vi "Writer data.vi"(8 "error in":errorcluster caption="错误输入（无错误）", 9 "数据输入":string[](array[string])=["TBOX", "7900020-CC102", "1", "1", "1", "2018/11/14 14:56:51 ", "1", "1", "1"], 11 "Slot":T1) -> (0 "error out":errorcluster caption="错误输出", 2 "Pass?":bool, 3 "添加的数组":string[][](array[string]))   [LabVIEW 2013]
uses:
  SystemCode/SysControl/Slot.ctl
  <vilib>/Utility/NIReport.llb/NI_report.lvclass
  <vilib>/addons/_office/excel.llb/Excel Get Data ([str]).vi
  <vilib>/addons/_office/excel.llb/Excel Easy Table (str).vi
  <vilib>/addons/_office/NI_ReportGenerationToolkit.lvlib
  <vilib>/Utility/NIReport.llb/Excel/NI_Excel.lvclass
panel:
  out "exists?":bool caption="文件或文件夹存在？"
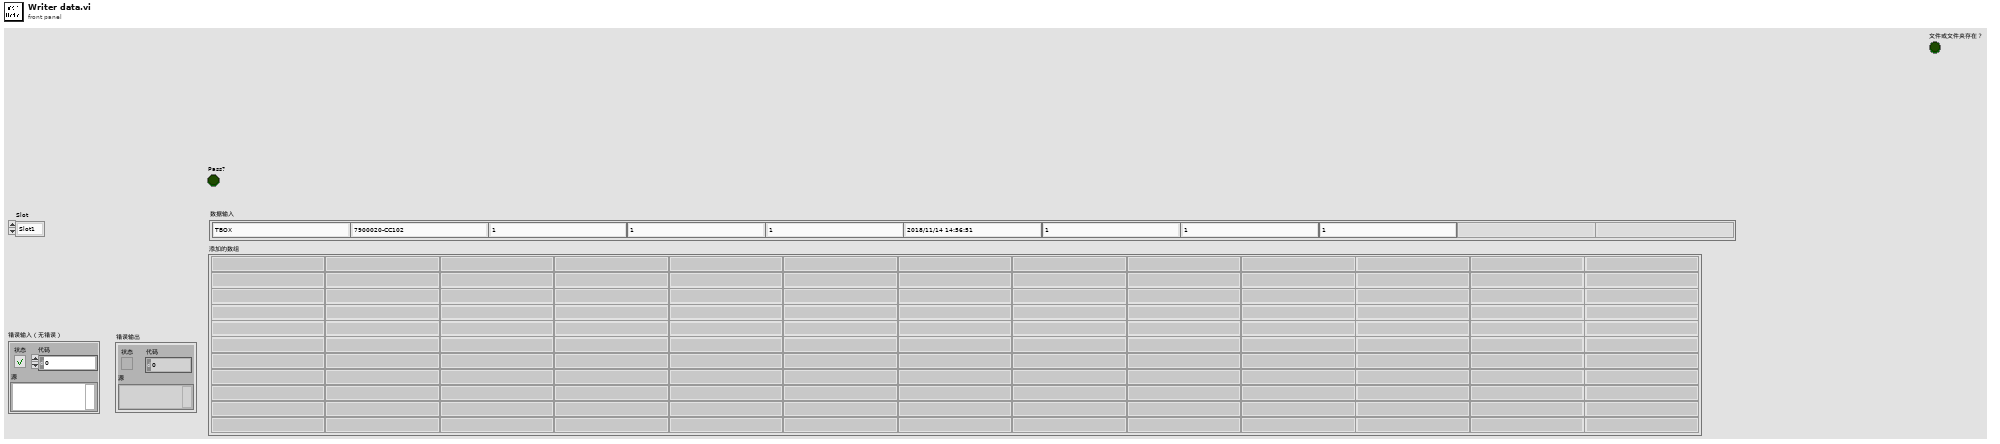
[diagram p1: front panel]
types:
  T1 = typedef "Slot.ctl" = enum16{"Slot1", "Slot2", "Slot3", "Slot4"}
  T2 = enum16{"Standard Report", "HTML", "Word", "Excel"}
  T3 = enum16{"maximized", "minimized", "normal", "no change"}
  T4 = enum32{"invalid app kind", "Development System", "Run Time System", "Student Edition", "Embedded LabVIEW", "Evaluation", "Custom"}
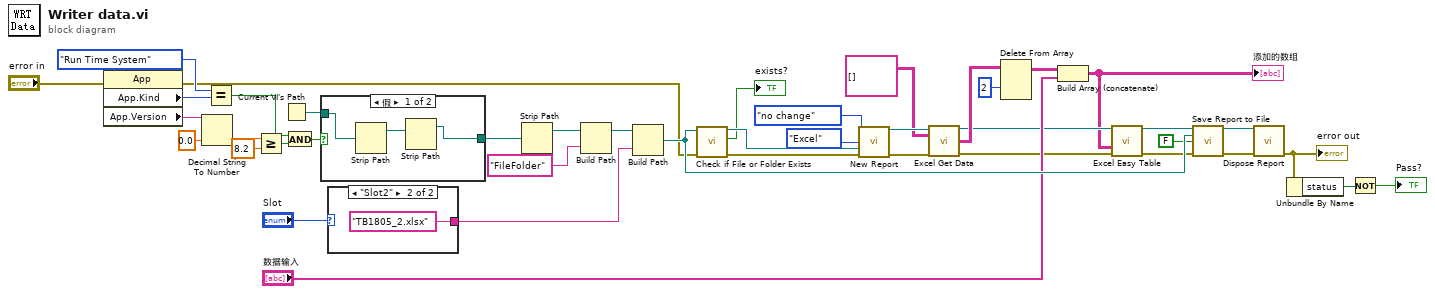
[diagram p0: block diagram]
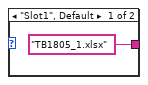
[diagram p2: hidden frame]
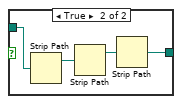
[diagram p3: hidden frame]
diagram:
  n1 = property class="App"(error in="error in") -> (error out=w4:errorcluster, "App.Kind"=w42:T4, "App.Version"=w40:string)  [unwired: 1 in, 1 out]
  n2 = Decimal String To Number(string=w40, default (0L)=0.0 ("数值")) -> (number=w39:dbl)  [unwired: 1 in, 1 out]
  n3 = Equal?(x=T4."Run Time System" ("应用程序:类别"), y=w42) -> (x = y?=w36:bool)
  n4 = Greater Or Equal?(x=w39, y=8.2) -> (x >= y?=w35:bool)
  n5 = Current VI's Path() -> (path=w33:path)
  n6 = And(x=w36, y=w35) -> (x .and. y?=w34:bool)
  n7 = case shown="假" w34 {
    tunnel: w33 -> [w45 w49]
    tunnel: [w43 w46] -> w32
    frame False {
      n8 = Strip Path(path=w45) -> (stripped path=w44:path)  [unwired: 1 out]
      n9 = Strip Path(path=w44) -> (stripped path=w43:path)  [unwired: 1 out]
    }
    frame True {
      n10 = Strip Path(path=w49) -> (stripped path=w48:path)  [unwired: 1 out]
      n11 = Strip Path(path=w48) -> (stripped path=w47:path)  [unwired: 1 out]
      n12 = Strip Path(path=w47) -> (stripped path=w46:path)  [unwired: 1 out]
    }
  }
  n13 = case shown="\"Slot2\"" "Slot" {
    tunnel: ["TB1805_1.xlsx" ("名称或相对路径") "TB1805_2.xlsx" ("名称或相对路径")] -> w8
    frame "Slot1", Default {
    }
    frame "Slot2" {
    }
  }
  n14 = Strip Path(path=w32) -> (stripped path=w31:path)  [unwired: 1 out]
  n15 = Build Path(base path=w31, name or relative path="FileFolder" ("名称或相对路径")) -> (appended path=w6:path)
  n16 = Build Path(base path=w6, name or relative path=w8) -> (appended path=w20:path)
  n17 = call <vilib>:"Check if File or Folder Exists.vi"("error in (no error)"=w4, "path"=w20) -> ("error out"=w27:errorcluster, "file or folder exists?"=→"exists?":bool, "dup path"=w30:path)  [unwired: 7 in]
  n18 = call <vilib>:"New Report.vi"("window state (normal)"=T3."no change", "report type"=T2."Excel", "template (empty)"=w30, "error in (no error)"=w27) -> ("report out"=w26:refnum<class "NI_report.lvclass">, "error out"=w25:errorcluster)  [unwired: 10 in]
  n19 = call-poly <vilib>:"Excel Get Data.vi"("report in"=w26, "data type"=string[][] [] ("数组"), "error in (no error)"=w25) -> ("report out"=w13:refnum<class "NI_report.lvclass">, "data"=w18:string[][], "error out"=w15:errorcluster)  [unwired: 10 in]
  n20 = Delete From Array(array=w18, index (row)=2 ("索引 (行)")) -> (array with subset deleted=w10:string[][])  [unwired: 2 in, 1 out]
  n21 = Build Array (concatenate)(w10, "数据输入") -> (w11:string[][])
  "添加的数组" <- w11
  n22 = call-poly <vilib>:"Excel Easy Table.vi"("report in"=w13, "text data"=w11, "error in (no error)"=w15) -> ("report out"=w12:refnum<class "NI_report.lvclass">, "error out"=w14:errorcluster)  [unwired: 8 in, 3 out]
  n23 = call-dynamic "Save Report to File.vi"("report in"=w12, "report file path"=w20, "prompt to replace? (F)"=FALSE, "error in (no error)"=w14) -> ("report out"=w21:refnum<class "NI_report.lvclass">, "error out"=w22:errorcluster)  [unwired: 10 in]
  n24 = call-dynamic "Dispose Report.vi"("report in"=w21, "error in (no error)"=w22) -> ("error out"=w3:errorcluster)  [unwired: 13 in]
  "error out" <- w3
  n25 = Unbundle By Name(w3) -> ("status"=w2:bool)
  n26 = Not(x=w2) -> (.not. x?=→"Pass?":bool)
